vi "quadrocopter.vi"() -> ()   [LabVIEW 2012]
panel:
  in  "-":bool
  in  "+":bool
  out "Status Bluetooth":string
  in  "Szybkoœæ silnika":u8(slide) scale=0.0..100.0
  in  "Opcja":u8(slide) max=5 step=1 scale=0.0..5.0
  out "error out":errorcluster
  in  "stop":bool
  out "Nazwa Bluetooth":string
  in  "Limit czasu":i32=1000
  # "Zwiêksz /zmniejsz\nmoc przy Czekaj"
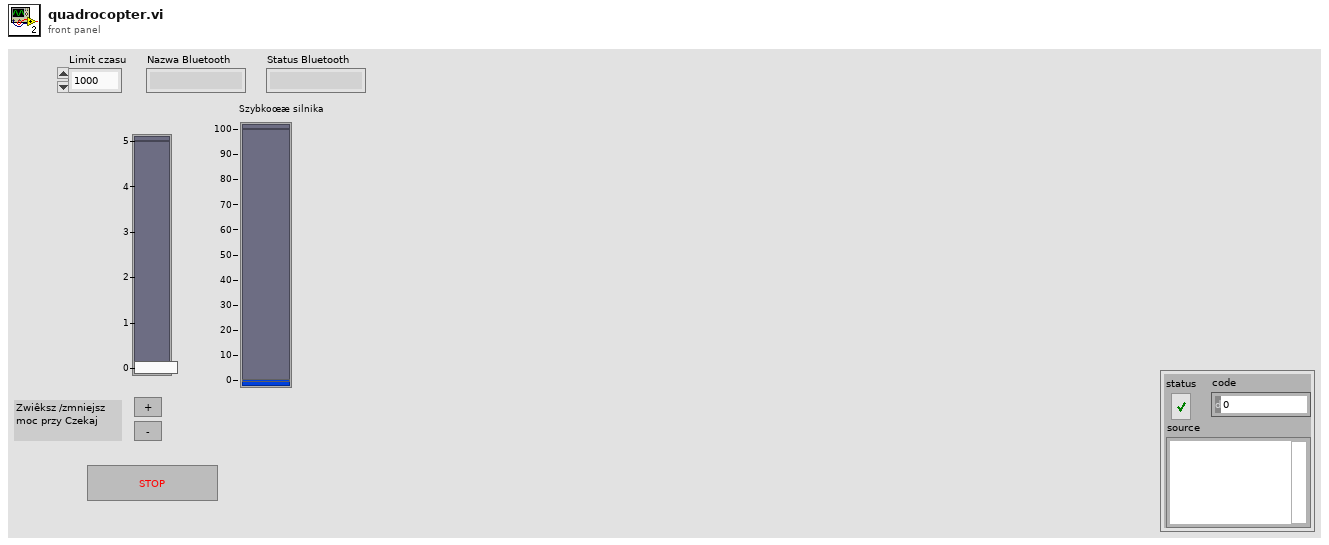
[diagram p1: front panel]
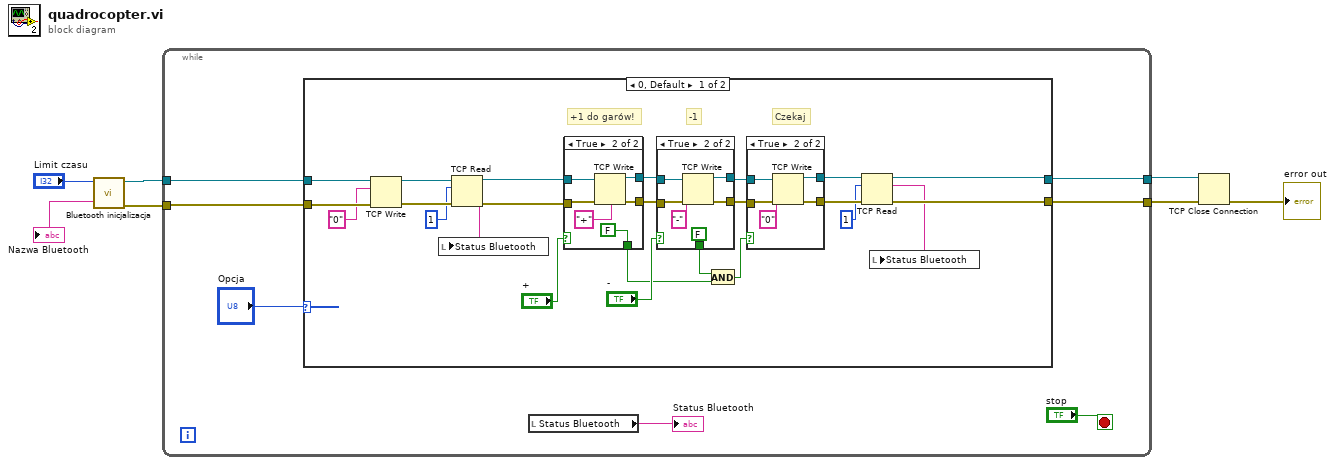
[diagram p0: block diagram]
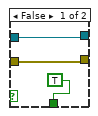
[diagram p3: hidden frame]
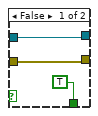
[diagram p4: hidden frame]
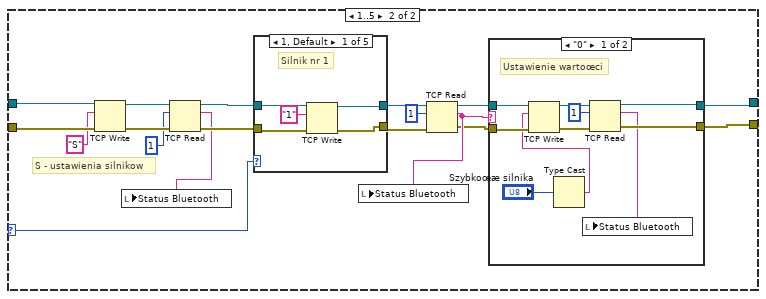
[diagram p5: hidden frame]
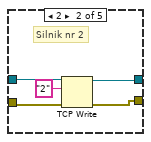
[diagram p7: hidden frame]
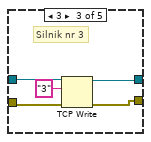
[diagram p8: hidden frame]
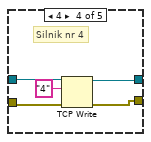
[diagram p9: hidden frame]
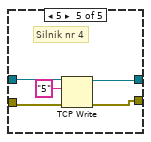
[diagram p10: hidden frame]
diagram:
  n1 = call "Bluetooth inicjalizacja.vi"("time limit ms (10000)"="Limit czasu") -> ("error out"=w2:errorcluster, "Bluetooth Network Connection out"=w4:refnum<k31>, "Device Name"=→"Nazwa Bluetooth":string)  [unwired: 5 in, 3 out]
  n2 = while {
    tunnel: [w10] -> w3
    tunnel: w4 -> [w12]
    tunnel: w2 -> [w11]
    tunnel: [w9] -> w1
    stop <- "stop" stop-if-true
    n3 = case shown="0, Default" "Opcja" {
      selector: "Opcja" -> [_ w72]
      tunnel: w12 -> [w38 w81]
      tunnel: w11 -> [w37 w80]
      tunnel: [w22 w66] -> w10
      tunnel: [w21 w65] -> w9
      frame 0, Default {
        # "Czekaj"
        # "-1"
        # "+1 do garów!"
        n4 = TCP Write(connection ID=w38, data in="0", error in (no error)=w37) -> (connection ID out=w35:refnum<k31>, error out=w34:errorcluster)  [unwired: 1 in, 1 out]
        n5 = TCP Read(connection ID=w35, bytes to read=1, error in (no error)=w34) -> (connection ID out=w31:refnum<k31>, data out=w32:string, error out=w30:errorcluster)  [unwired: 2 in]
        n6 = local write "Status Bluetooth"(w32) -> ()
        n7 = case shown="True" "+" {
          tunnel: w31 -> [w57 w63]
          tunnel: w30 -> [w56 w62]
          tunnel: [w56 w60] -> w29
          tunnel: [w57 w59] -> w28
          tunnel: [TRUE FALSE] -> w16
          frame False {
          }
          frame True {
            n8 = TCP Write(connection ID=w63, data in="+", error in (no error)=w62) -> (connection ID out=w59:refnum<k31>, error out=w60:errorcluster)  [unwired: 1 in, 1 out]
          }
        }
        n9 = case shown="True" "-" {
          tunnel: w28 -> [w48 w54]
          tunnel: w29 -> [w47 w53]
          tunnel: [w47 w51] -> w27
          tunnel: [w48 w50] -> w26
          tunnel: [TRUE FALSE] -> w15
          frame False {
          }
          frame True {
            n10 = TCP Write(connection ID=w54, data in="-", error in (no error)=w53) -> (connection ID out=w50:refnum<k31>, error out=w51:errorcluster)  [unwired: 1 in, 1 out]
          }
        }
        n11 = And(x=w15, y=w16) -> (x .and. y?=w17:bool)
        n12 = case shown="True" w17 {
          tunnel: w26 -> [w40 w45]
          tunnel: w27 -> [w39 w44]
          tunnel: [w39 w42] -> w24
          tunnel: [w40 w41] -> w25
          frame False {
          }
          frame True {
            n13 = TCP Write(connection ID=w45, data in="0", error in (no error)=w44) -> (connection ID out=w41:refnum<k31>, error out=w42:errorcluster)  [unwired: 1 in, 1 out]
          }
        }
        n14 = TCP Read(connection ID=w25, bytes to read=1, error in (no error)=w24) -> (connection ID out=w22:refnum<k31>, data out=w20:string, error out=w21:errorcluster)  [unwired: 2 in]
        n15 = local write "Status Bluetooth"(w20) -> ()
      }
      frame 1..5 {
        # "S - ustawienia silnikow"
        n16 = TCP Write(connection ID=w81, data in="S", error in (no error)=w80) -> (connection ID out=w77:refnum<k31>, error out=w78:errorcluster)  [unwired: 1 in, 1 out]
        n17 = TCP Read(connection ID=w77, bytes to read=1, error in (no error)=w78) -> (connection ID out=w74:refnum<k31>, data out=w73:string, error out=w75:errorcluster)  [unwired: 2 in]
        n18 = local write "Status Bluetooth"(w73) -> ()
        n19 = case shown="1, Default" w72 {
          tunnel: w75 -> [w97 w102 w107 w112 w117]
          tunnel: w74 -> [w98 w103 w108 w113 w118]
          tunnel: [w95 w100 w105 w110 w115] -> w71
          tunnel: [w94 w99 w104 w109 w114] -> w70
          frame 1, Default {
            # "Silnik nr 1"
            n20 = TCP Write(connection ID=w98, data in="1", error in (no error)=w97) -> (connection ID out=w95:refnum<k31>, error out=w94:errorcluster)  [unwired: 1 in, 1 out]
          }
          frame 2 {
            # "Silnik nr 2"
            n21 = TCP Write(connection ID=w103, data in="2", error in (no error)=w102) -> (connection ID out=w100:refnum<k31>, error out=w99:errorcluster)  [unwired: 1 in, 1 out]
          }
          frame 3 {
            # "Silnik nr 3"
            n22 = TCP Write(connection ID=w108, data in="3", error in (no error)=w107) -> (connection ID out=w105:refnum<k31>, error out=w104:errorcluster)  [unwired: 1 in, 1 out]
          }
          frame 4 {
            # "Silnik nr 4"
            n23 = TCP Write(connection ID=w113, data in="4", error in (no error)=w112) -> (connection ID out=w110:refnum<k31>, error out=w109:errorcluster)  [unwired: 1 in, 1 out]
          }
          frame 5 {
            # "Silnik nr 4"
            n24 = TCP Write(connection ID=w118, data in="5", error in (no error)=w117) -> (connection ID out=w115:refnum<k31>, error out=w114:errorcluster)  [unwired: 1 in, 1 out]
          }
        }
        n25 = TCP Read(connection ID=w71, bytes to read=1, error in (no error)=w70) -> (connection ID out=w67:refnum<k31>, data out=w68:string, error out=w64:errorcluster)  [unwired: 2 in]
        n26 = local write "Status Bluetooth"(w68) -> ()
        n27 = case shown="\"0\"" w68 {
          tunnel: [w85 w93] -> w66
          tunnel: w67 -> [w91 w93]
          tunnel: [w84 w92] -> w65
          tunnel: w64 -> [w90 w92]
          frame "0" {
            # "Ustawienie wartoœci"
            n28 = Type Cast(x="Szybkoœæ silnika") -> (*(type *) &x=w88:string)  [unwired: 1 in]
            n29 = TCP Write(connection ID=w91, data in=w88, error in (no error)=w90) -> (connection ID out=w87:refnum<k31>, error out=w86:errorcluster)  [unwired: 1 in, 1 out]
            n30 = TCP Read(connection ID=w87, bytes to read=1, error in (no error)=w86) -> (connection ID out=w85:refnum<k31>, data out=w83:string, error out=w84:errorcluster)  [unwired: 2 in]
            n31 = local write "Status Bluetooth"(w83) -> ()
          }
          frame "1", Default {
          }
        }
      }
    }
    n32 = local read "Status Bluetooth"() -> (→"Status Bluetooth":string)
  }
  n33 = TCP Close Connection(connection ID=w3, error in (no error)=w1) -> (error out=→"error out":errorcluster)  [unwired: 1 in, 1 out]
